vi "DirectionCommandDelay.vi"(3 "Motor PWM Request":dbl, 4 "Current Direction":bool, 5 "Direction Request":bool) -> (0 "Motor PWM Command":dbl, 1 "Direction Enabled":bool caption="Time has Elapsed", 2 "Direction Command":bool)   [LabVIEW 2013]
panel:
  out "Elapsed Time (s)":dbl
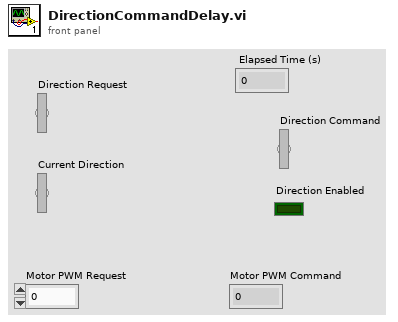
[diagram p1: front panel]
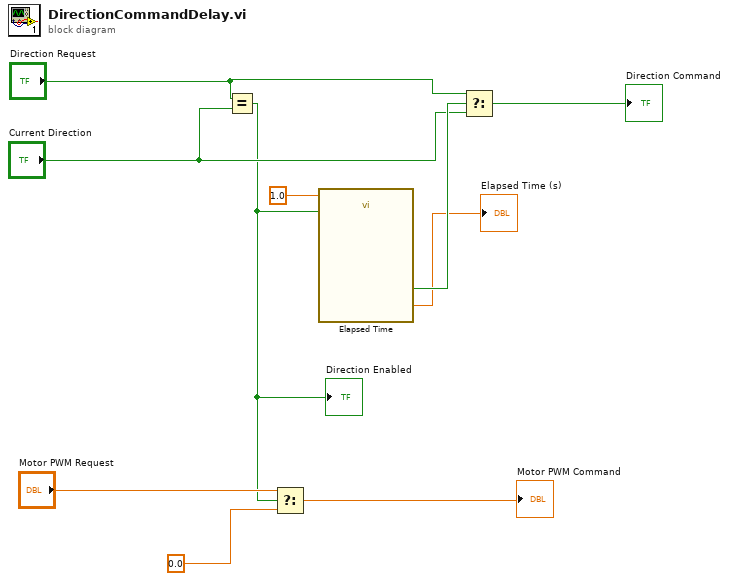
[diagram p0: block diagram]
diagram:
  n1 = Equal?(x="Direction Request", y="Current Direction") -> (x = y?=w1:bool)
  "Direction Enabled" <- w1
  n2 = Select(t="Motor PWM Request", s=w1, f=0.0) -> (s? t:f=→"Motor PWM Command":dbl)
  n3 = call "Elapsed Time"("Time Target (s)"=1.0, "Reset"=w1) -> ("Elapsed Time (s)"=→"Elapsed Time (s)":dbl, "Time has Elapsed"=w8:bool)  [unwired: 10 in, 6 out]
  n4 = Select(t="Direction Request", s=w8, f="Current Direction") -> (s? t:f=→"Direction Command":bool)
